vi "GetSwerveEncoders.vi"() -> (16 "Swerve 0 Velocity (ft/s)":dbl, 17 "Swerve 3 Velocity (ft/s)":dbl, 18 "Swerve 1 Velocity (ft/s)":dbl, 19 "Swerve 2 Velocity (ft/s)":dbl, 20 "Swerve 0 Azimuth Position (deg)":dbl, 21 "Swerve 0 Distance (in)":dbl, 22 "Swerve 1 Azimuth Position (deg)":dbl, 23 "Swerve 1 Distance (in)":dbl, 24 "Swerve 2 Azimuth Position (deg)":dbl, 25 "Swerve 2 Distance (in)":dbl, 26 "Swerve 3 Azimuth Position (deg)":dbl, 27 "Swerve 3 Distance (in)":dbl)   [LabVIEW 2019]
doc: "Gets the drive distance, azimuth position, and velocity encoder readings from all of the swerve modules. This VI is also useful for characterizing the drive system allowing for estimation of the robot acceleration and plotting of the module velocities. Deteremines the true shifter state based on photo-interrupter sensors on each module. Please see sensors.vi for a reading of the true robot ground speed (as this must be calculated after using the module odometry VIs)."
uses:
  9b416838-22f8-4a95-87d5-07d0cb0d5b1f.vi
  refnums.vi
  GRNF_POT.vi
  dsdata.vi
  <vilib>/Utility/xml.llb/Write to XML File(string).vi
  GRNF_CTREMotor.vi
  <vilib>/Rock Robotics/WPI/ThirdParty/Phoenix-LabVIEW/Motor Controller/Get/CTRE_Phoenix_MotorController_GetSelectedSensorData.vi
  GRNF_DI.vi
  sensors.vi
panel:
  out "Current Position (deg)":dbl
  in  "Calibrate Lamprey":T1(ring)
  out "Within Tolerance":bool
  out "Calibration Goal (deg) [0,360]":dbl format="%.2f"
  in  "Lamprey Tolerance (deg)":dbl=0.1
  in  "Calibration Step":i16
  in  "Calibration Mode":T2(ring)
  in  "Set Falcon Zero":bool
  out "Acceleration (ft/s^2)":dbl format="%.1f"
  in  "Reset Acceleration Test":bool
  in  "Plot and Measure":bool
  out "Drive Encoder Velocities (ft/s)":cluster{dbl, dbl, dbl, dbl}(graph)
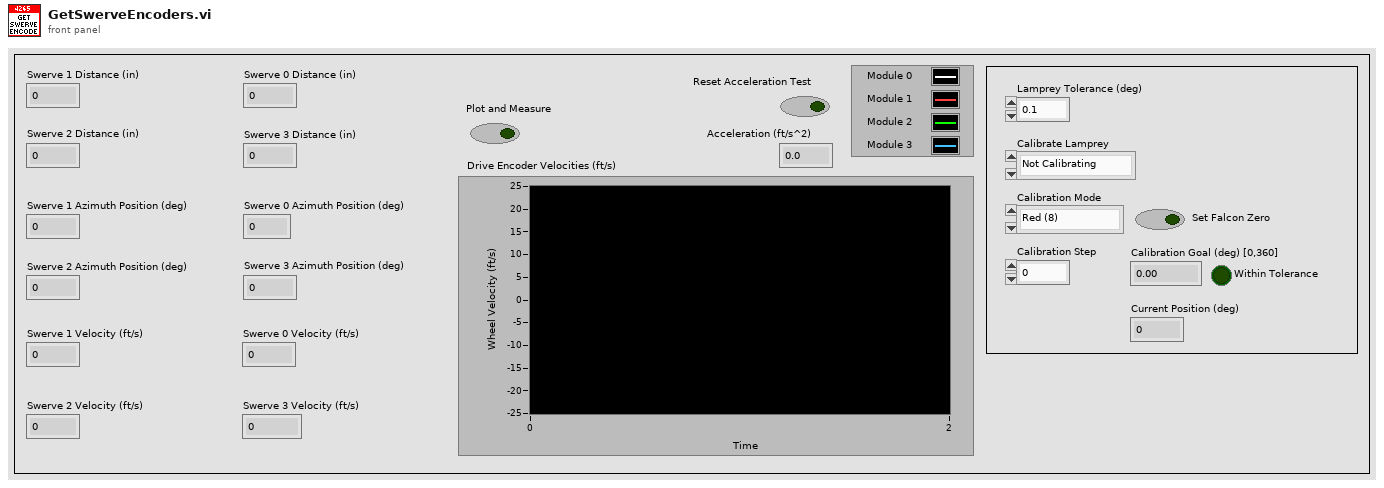
[diagram p1: front panel]
types:
  T1 = enum16{"Not Calibrating", "Module 0", "Module 1", "Module 2", "Module 3"}
  T2 = enum16{"Red (8)", "Red+Green (12)", "Red+Green+Blue (24)", "Blue (36)"}
  T3 = typedef "WPI_SwitchDevRef.ctl" = cluster{"DevStatus":errorcluster, "DIO Channel":T4, "CntIndex":T5, "Normally Closed":bool}
  T4 = typedef "FPGA_DIOChannel.ctl" = enum8{"DIO 0", "DIO 1", "DIO 2", "DIO 3", "DIO 4", "DIO 5", "DIO 6", "DIO 7", "DIO 8", "DIO 9", "DIO MXP 0", "DIO MXP 1", "DIO MXP 2", "DIO MXP 3", "DIO MXP 4", "DIO MXP 5", "DIO MXP 6", "DIO MXP 7", "DIO MXP 8", "DIO MXP 9", "DIO MXP 10", "DIO MXP 11", "DIO MXP 12", "DIO MXP 13", "DIO MXP 14", "DIO MXP 15", "SPI Port CS1", "SPI Port CS2", "SPI Port CS3", "SPI Port MISO", "SPI Port MOSI", "Invalid"}
  T5 = typedef "FPGA_CounterCtrSystemIndex.ctl" = enum8{"Ctr 0", "Ctr 1", "Ctr 2", "Ctr 3", "Ctr 4", "Ctr 5", "Ctr 6", "Ctr 7", "Invalid"}
  T6 = enum16{"Low Gear", "High Gear", "Transiting", "Unknown", "Force Low Gear"}
  T7 = typedef "WPI_MotorControlDeviceRef.ctl" = cluster{"DeviceStatus":errorcluster, "Type":T8, "PWM":cluster{"PWM Channel":T9, "DeadBand":T10}, "CAN":cluster{"Device Number":u8, "SetOutput VI Ref":variant, "GetOutput VI Ref":variant, "Enable VI Ref":variant, "Disable VI Ref":variant, "Data":variant}, "Invert":bool, "DIO PWM":cluster{"PWM \"Enable\" Channel":T9, "DIOChannel":T4, "PWM Rate":dbl}}
  T8 = typedef "WPI_MotorControlType.ctl" = enum16{"PWM", "CAN", "DIO PWM"}
  T9 = typedef "FPGA_DIOPWMChannel.ctl" = enum8{"PWM 0", "PWM 1", "PWM 2", "PWM 3", "PWM 4", "PWM 5", "PWM 6", "PWM 7", "PWM 8", "PWM 9", "PWM MXP 0", "PWM MXP 1", "PWM MXP 2", "PWM MXP 3", "PWM MXP 4", "PWM MXP 5", "PWM MXP 6", "PWM MXP 7", "PWM MXP 8", "PWM MXP 9", "Invalid"}
  T10 = typedef "WPI_PWMDeadband.ctl" = cluster{"Name":string, "maxPositivePwm":i32, "minPositivePwm":i32, "centerPwm":i32, "maxNegativePwm":i32, "minNegativePwm":i32, "angularRange":u16}
  T11 = typedef "WPI_PotentiometerDevRef.ctl" = cluster{"DevStatus":errorcluster, "Analog Channel":T12, "Invert Output":bool}
  T12 = typedef "FPGA_AIChannel.ctl" = enum8{"AI 0", "AI 1", "AI 2", "AI 3", "AI MXP 0", "AI MXP 1", "AI MXP 2", "AI MXP 3", "Invalid"}
  T13 = cluster{"Velocity (ft/s)":dbl, "Velocity (ft/s)":dbl, "Velocity (ft/s)":dbl, "Velocity (ft/s)":dbl}
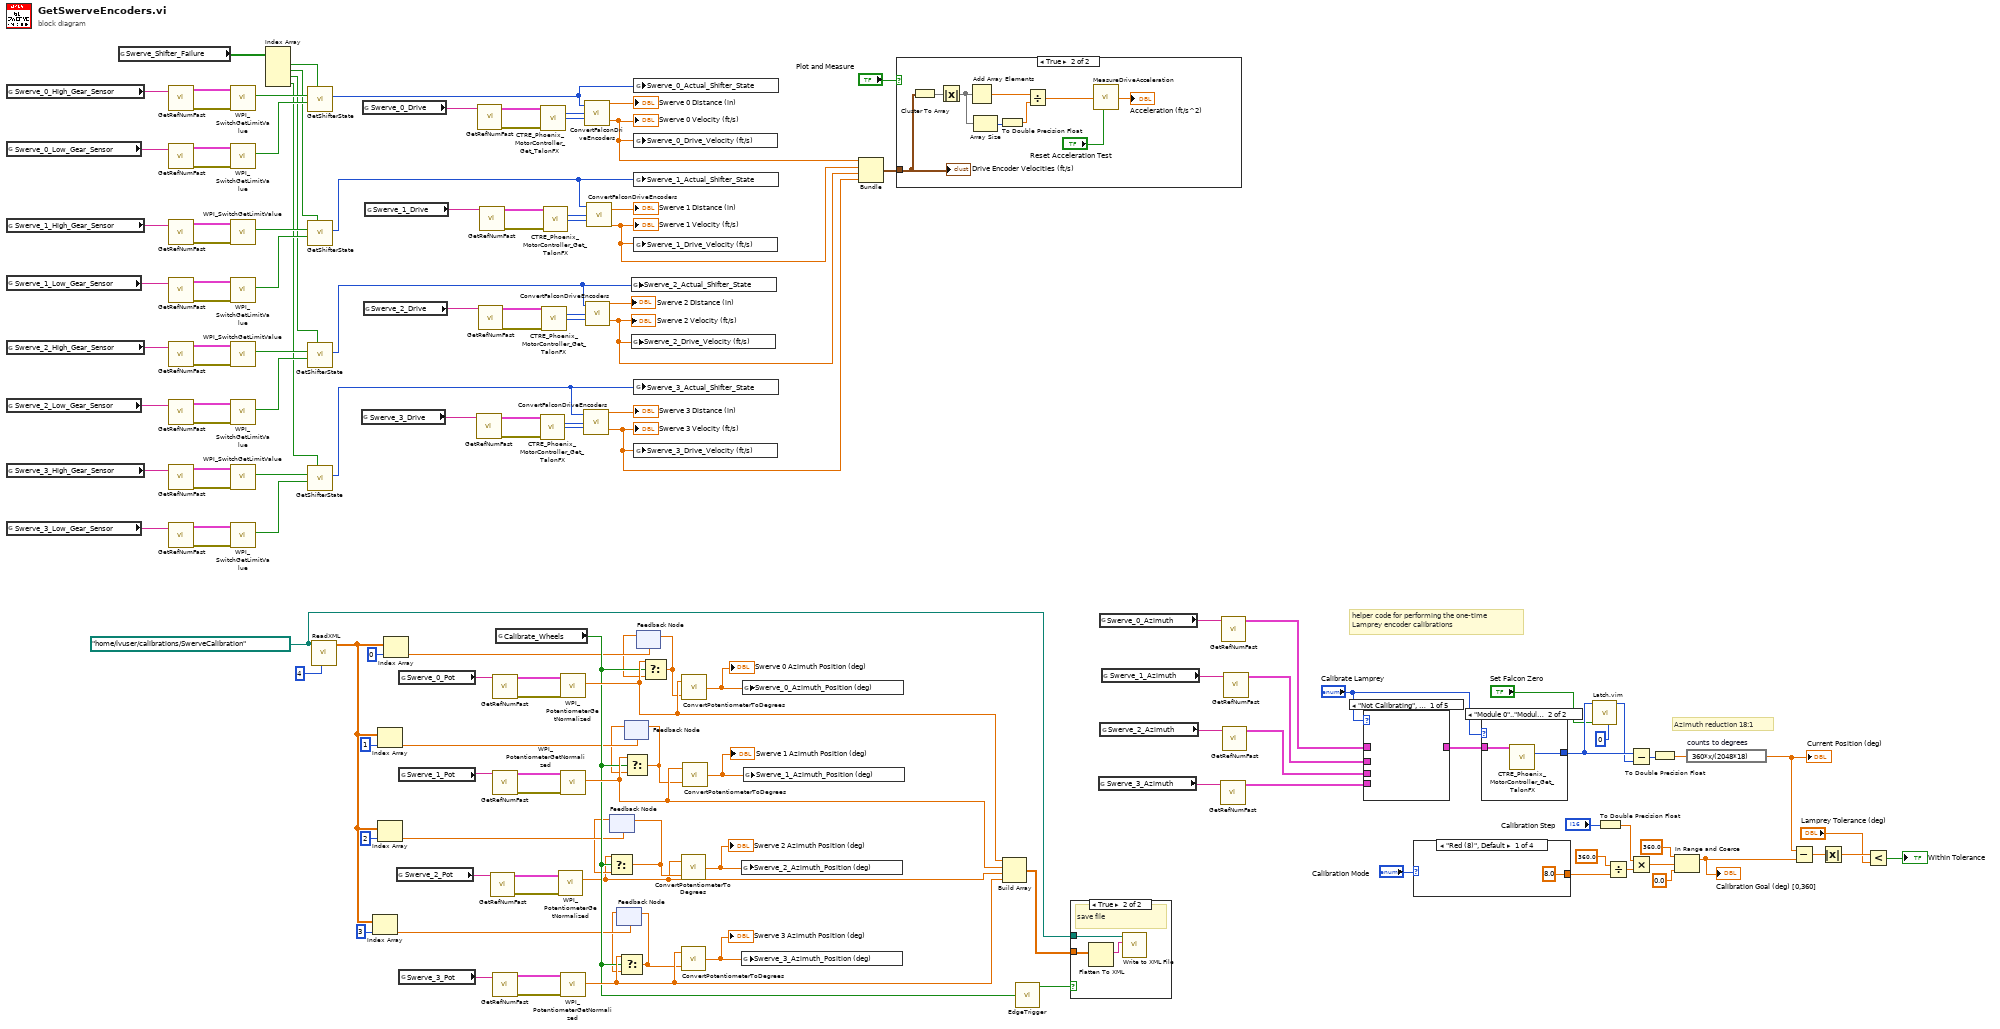
[diagram p0: block diagram]
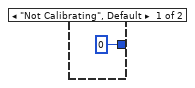
[diagram p6: hidden frame]
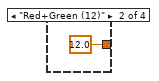
[diagram p7: hidden frame]
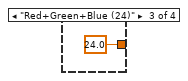
[diagram p8: hidden frame]
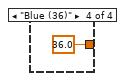
[diagram p9: hidden frame]
diagram:
  w140 = path "/home/lvuser/calibrations/SwerveCalibration" ("path")
  # "Azimuth reduction 18:1"
  # "helper code for performing the one-time\nLamprey encoder calibrations"
  n1 = global read "refnums.vi" "Swerve_0_High_Gear_Sensor"() -> (w44:string)
  n2 = global read "refnums.vi" "Swerve_0_Low_Gear_Sensor"() -> (w40:string)
  n3 = global read "refnums.vi" "Swerve_1_High_Gear_Sensor"() -> (w36:string)
  n4 = global read "refnums.vi" "Swerve_1_Low_Gear_Sensor"() -> (w32:string)
  n5 = global read "refnums.vi" "Swerve_2_High_Gear_Sensor"() -> (w27:string)
  n6 = global read "refnums.vi" "Swerve_2_Low_Gear_Sensor"() -> (w23:string)
  n7 = global read "refnums.vi" "Swerve_3_High_Gear_Sensor"() -> (w18:string)
  n8 = global read "refnums.vi" "Swerve_3_Low_Gear_Sensor"() -> (w14:string)
  n9 = global read "sensors.vi" "Swerve_Shifter_Failure"() -> (w9:bool[])
  n10 = call-poly "GetRefNumFast.vi"("RefNum Name"=w44) -> ("Error"=w42:errorcluster, "Device Reference"=w43:T3)  [unwired: 5 in]
  n11 = call-poly "GetRefNumFast.vi"("RefNum Name"=w40) -> ("Error"=w38:errorcluster, "Device Reference"=w39:T3)  [unwired: 5 in]
  n12 = call-poly "GetRefNumFast.vi"("RefNum Name"=w36) -> ("Error"=w34:errorcluster, "Device Reference"=w35:T3)  [unwired: 5 in]
  n13 = call-poly "GetRefNumFast.vi"("RefNum Name"=w32) -> ("Error"=w30:errorcluster, "Device Reference"=w31:T3)  [unwired: 5 in]
  n14 = call-poly "GetRefNumFast.vi"("RefNum Name"=w27) -> ("Error"=w25:errorcluster, "Device Reference"=w26:T3)  [unwired: 5 in]
  n15 = call-poly "GetRefNumFast.vi"("RefNum Name"=w23) -> ("Error"=w21:errorcluster, "Device Reference"=w22:T3)  [unwired: 5 in]
  n16 = call-poly "GetRefNumFast.vi"("RefNum Name"=w18) -> ("Error"=w16:errorcluster, "Device Reference"=w17:T3)  [unwired: 5 in]
  n17 = call-poly "GetRefNumFast.vi"("RefNum Name"=w14) -> ("Error"=w12:errorcluster, "Device Reference"=w13:T3)  [unwired: 5 in]
  n18 = call <vilib>:"WPI_SwitchGetLimitValue.vi"("error in (no error)"=w42, "SwitchDevRef"=w43) -> ("Switch Pressed"=w41:bool)  [unwired: 7 in, 2 out]
  n19 = call <vilib>:"WPI_SwitchGetLimitValue.vi"("error in (no error)"=w38, "SwitchDevRef"=w39) -> ("Switch Pressed"=w37:bool)  [unwired: 7 in, 2 out]
  n20 = call <vilib>:"WPI_SwitchGetLimitValue.vi"("error in (no error)"=w34, "SwitchDevRef"=w35) -> ("Switch Pressed"=w33:bool)  [unwired: 7 in, 2 out]
  n21 = call <vilib>:"WPI_SwitchGetLimitValue.vi"("error in (no error)"=w30, "SwitchDevRef"=w31) -> ("Switch Pressed"=w29:bool)  [unwired: 7 in, 2 out]
  n22 = call <vilib>:"WPI_SwitchGetLimitValue.vi"("error in (no error)"=w25, "SwitchDevRef"=w26) -> ("Switch Pressed"=w24:bool)  [unwired: 7 in, 2 out]
  n23 = call <vilib>:"WPI_SwitchGetLimitValue.vi"("error in (no error)"=w21, "SwitchDevRef"=w22) -> ("Switch Pressed"=w20:bool)  [unwired: 7 in, 2 out]
  n24 = call <vilib>:"WPI_SwitchGetLimitValue.vi"("error in (no error)"=w16, "SwitchDevRef"=w17) -> ("Switch Pressed"=w15:bool)  [unwired: 7 in, 2 out]
  n25 = call <vilib>:"WPI_SwitchGetLimitValue.vi"("error in (no error)"=w12, "SwitchDevRef"=w13) -> ("Switch Pressed"=w11:bool)  [unwired: 7 in, 2 out]
  n26 = Index Array(array=w9) -> (element #1=w8:bool, element #2=w7:bool, element #3=w6:bool, element #4=w5:bool)  [unwired: 4 in]
  n27 = call "GetShifterState.vi"("Sensor Failure"=w8, "Low Gear Sensor"=w37, "High Gear Sensor"=w41) -> ("Actual Shifter State"=w45:T6)  [unwired: 8 in]
  n28 = call "GetShifterState.vi"("Sensor Failure"=w7, "Low Gear Sensor"=w29, "High Gear Sensor"=w33) -> ("Actual Shifter State"=w28:T6)  [unwired: 8 in]
  n29 = call "GetShifterState.vi"("Sensor Failure"=w6, "Low Gear Sensor"=w20, "High Gear Sensor"=w24) -> ("Actual Shifter State"=w19:T6)  [unwired: 8 in]
  n30 = call "GetShifterState.vi"("Sensor Failure"=w5, "Low Gear Sensor"=w11, "High Gear Sensor"=w15) -> ("Actual Shifter State"=w10:T6)  [unwired: 8 in]
  n31 = call "ReadXML.vi"("Default Number of Elements"=4 ("Number of Elements"), "File Path (.xml)"=w140) -> ("Data"=w106:dbl[])  [unwired: 8 in, 1 out]
  n32 = global read "refnums.vi" "Swerve_3_Drive"() -> (w81:string)
  n33 = global read "refnums.vi" "Swerve_0_Drive"() -> (w101:string)
  n34 = global read "refnums.vi" "Swerve_2_Drive"() -> (w88:string)
  n35 = global read "refnums.vi" "Swerve_1_Drive"() -> (w93:string)
  n36 = Index Array(array=w106, index=3) -> (element=w124:dbl)
  n37 = Index Array(array=w106, index=1) -> (element=w129:dbl)
  n38 = Index Array(array=w106, index=2) -> (element=w126:dbl)
  n39 = Index Array(array=w106, index=0) -> (element=w132:dbl)
  n40 = global read "refnums.vi" "Swerve_2_Pot"() -> (w110:string)
  n41 = global read "refnums.vi" "Swerve_0_Pot"() -> (w118:string)
  n42 = global read "refnums.vi" "Swerve_1_Pot"() -> (w113:string)
  n43 = global read "refnums.vi" "Swerve_3_Pot"() -> (w109:string)
  n44 = call-poly "GetRefNumFast.vi"("RefNum Name"=w81) -> ("Error"=w83:errorcluster, "Device Reference"=w82:T7)  [unwired: 5 in]
  n45 = call-poly "GetRefNumFast.vi"("RefNum Name"=w101) -> ("Error"=w103:errorcluster, "Device Reference"=w102:T7)  [unwired: 5 in]
  n46 = call-poly "GetRefNumFast.vi"("RefNum Name"=w88) -> ("Error"=w2:errorcluster, "Device Reference"=w1:T7)  [unwired: 5 in]
  n47 = call-poly "GetRefNumFast.vi"("RefNum Name"=w93) -> ("Error"=w95:errorcluster, "Device Reference"=w94:T7)  [unwired: 5 in]
  n48 = call-poly "GetRefNumFast.vi"("RefNum Name"=w110) -> ("Error"=w111:errorcluster, "Device Reference"=w112:T11)  [unwired: 5 in]
  n49 = call-poly "GetRefNumFast.vi"("RefNum Name"=w118) -> ("Error"=w116:errorcluster, "Device Reference"=w117:T11)  [unwired: 5 in]
  n50 = call-poly "GetRefNumFast.vi"("RefNum Name"=w113) -> ("Error"=w114:errorcluster, "Device Reference"=w115:T11)  [unwired: 5 in]
  n51 = call-poly "GetRefNumFast.vi"("RefNum Name"=w109) -> ("Error"=w107:errorcluster, "Device Reference"=w108:T11)  [unwired: 5 in]
  n52 = global read "dsdata.vi" "Calibrate_Wheels"() -> (w139:bool)
  n53 = call-poly <vilib>:"CTRE_Phoenix_MotorController_Get_TalonFX.vi"("PhoenixMotorControlDevRef"=w82, "error in"=w83) -> ("Position (Raw Sensor Units)"=w79:i32, "Velocity (Raw Sensor Units per 100 ms)"=w80:i32)  [unwired: 10 in, 2 out]
  n54 = call-poly <vilib>:"CTRE_Phoenix_MotorController_Get_TalonFX.vi"("PhoenixMotorControlDevRef"=w102, "error in"=w103) -> ("Position (Raw Sensor Units)"=w96:i32, "Velocity (Raw Sensor Units per 100 ms)"=w97:i32)  [unwired: 10 in, 2 out]
  n55 = call-poly <vilib>:"CTRE_Phoenix_MotorController_Get_TalonFX.vi"("PhoenixMotorControlDevRef"=w1, "error in"=w2) -> ("Position (Raw Sensor Units)"=w86:i32, "Velocity (Raw Sensor Units per 100 ms)"=w87:i32)  [unwired: 10 in, 2 out]
  n56 = call-poly <vilib>:"CTRE_Phoenix_MotorController_Get_TalonFX.vi"("PhoenixMotorControlDevRef"=w94, "error in"=w95) -> ("Position (Raw Sensor Units)"=w91:i32, "Velocity (Raw Sensor Units per 100 ms)"=w92:i32)  [unwired: 10 in, 2 out]
  n57 = call <vilib>:"WPI_PotentiometerGetNormalized.vi"("error in"=w111, "PotDevRef"=w112) -> ("Normalized Value"=w3:dbl)  [unwired: 7 in, 2 out]
  n58 = call <vilib>:"WPI_PotentiometerGetNormalized.vi"("error in"=w116, "PotDevRef"=w117) -> ("Normalized Value"=w141:dbl)  [unwired: 7 in, 2 out]
  n59 = call <vilib>:"WPI_PotentiometerGetNormalized.vi"("error in"=w114, "PotDevRef"=w115) -> ("Normalized Value"=w143:dbl)  [unwired: 7 in, 2 out]
  n60 = call <vilib>:"WPI_PotentiometerGetNormalized.vi"("error in"=w107, "PotDevRef"=w108) -> ("Normalized Value"=w142:dbl)  [unwired: 7 in, 2 out]
  n61 = call "ConvertFalconDriveEncoders.vi"("Velocity (Raw Sensor Units per 100 ms)"=w80, "Distance (Raw Sensor Units)"=w79, "Shifter State"=w10) -> ("Velocity (ft/s)"=w77:dbl, "Distance (in)"=→"Swerve 3 Distance (in)":dbl)
  "Swerve 3 Velocity (ft/s)" <- w77
  n62 = call "ConvertFalconDriveEncoders.vi"("Velocity (Raw Sensor Units per 100 ms)"=w97, "Distance (Raw Sensor Units)"=w96, "Shifter State"=w45) -> ("Velocity (ft/s)"=w99:dbl, "Distance (in)"=→"Swerve 0 Distance (in)":dbl)
  "Swerve 0 Velocity (ft/s)" <- w99
  n63 = call "ConvertFalconDriveEncoders.vi"("Velocity (Raw Sensor Units per 100 ms)"=w87, "Distance (Raw Sensor Units)"=w86, "Shifter State"=w19) -> ("Velocity (ft/s)"=w84:dbl, "Distance (in)"=→"Swerve 2 Distance (in)":dbl)
  "Swerve 2 Velocity (ft/s)" <- w84
  n64 = call "ConvertFalconDriveEncoders.vi"("Velocity (Raw Sensor Units per 100 ms)"=w92, "Distance (Raw Sensor Units)"=w91, "Shifter State"=w28) -> ("Velocity (ft/s)"=w89:dbl, "Distance (in)"=→"Swerve 1 Distance (in)":dbl)
  "Swerve 1 Velocity (ft/s)" <- w89
  n65 = feedback #1(w126) -> (w125:dbl)
  n66 = Select(t=w3, s=w139, f=w125) -> (s? t:f=w4:dbl)
  n67 = feedback-in #1(w4) -> ()
  n68 = feedback #2(w124) -> (w123:dbl)
  n69 = Select(t=w142, s=w139, f=w123) -> (s? t:f=w119:dbl)
  n70 = feedback-in #2(w119) -> ()
  n71 = feedback #3(w129) -> (w128:dbl)
  n72 = Select(t=w143, s=w139, f=w128) -> (s? t:f=w120:dbl)
  n73 = feedback-in #3(w120) -> ()
  n74 = global write "sensors.vi" "Swerve_2_Actual_Shifter_State"(w19) -> ()
  n75 = global write "sensors.vi" "Swerve_2_Drive_Velocity (ft/s)"(w84) -> ()
  n76 = global write "sensors.vi" "Swerve_0_Actual_Shifter_State"(w45) -> ()
  n77 = global write "sensors.vi" "Swerve_0_Drive_Velocity (ft/s)"(w99) -> ()
  n78 = global write "sensors.vi" "Swerve_1_Actual_Shifter_State"(w28) -> ()
  n79 = global write "sensors.vi" "Swerve_1_Drive_Velocity (ft/s)"(w89) -> ()
  n80 = global write "sensors.vi" "Swerve_3_Actual_Shifter_State"(w10) -> ()
  n81 = global write "sensors.vi" "Swerve_3_Drive_Velocity (ft/s)"(w77) -> ()
  n82 = feedback #4(w132) -> (w131:dbl)
  n83 = Select(t=w141, s=w139, f=w131) -> (s? t:f=w121:dbl)
  n84 = feedback-in #4(w121) -> ()
  n85 = call "ConvertPotentiometerToDegrees.vi"("Zero Position [0-1]"=w4, "Raw Potentiometer Value [0,1]"=w3) -> ("Orientation (deg) [-180,+180]"=w135:dbl)
  "Swerve 2 Azimuth Position (deg)" <- w135
  n86 = call "ConvertPotentiometerToDegrees.vi"("Zero Position [0-1]"=w119, "Raw Potentiometer Value [0,1]"=w142) -> ("Orientation (deg) [-180,+180]"=w134:dbl)
  "Swerve 3 Azimuth Position (deg)" <- w134
  n87 = call "ConvertPotentiometerToDegrees.vi"("Zero Position [0-1]"=w121, "Raw Potentiometer Value [0,1]"=w141) -> ("Orientation (deg) [-180,+180]"=w137:dbl)
  "Swerve 0 Azimuth Position (deg)" <- w137
  n88 = call "ConvertPotentiometerToDegrees.vi"("Zero Position [0-1]"=w120, "Raw Potentiometer Value [0,1]"=w143) -> ("Orientation (deg) [-180,+180]"=w136:dbl)
  "Swerve 1 Azimuth Position (deg)" <- w136
  n89 = global write "sensors.vi" "Swerve_2_Azimuth_Position (deg)"(w135) -> ()
  n90 = global write "sensors.vi" "Swerve_3_Azimuth_Position (deg)"(w134) -> ()
  n91 = global write "sensors.vi" "Swerve_0_Azimuth_Position (deg)"(w137) -> ()
  n92 = global write "sensors.vi" "Swerve_1_Azimuth_Position (deg)"(w136) -> ()
  n93 = Bundle("Velocity (ft/s)"=w99, "Velocity (ft/s)"=w89, "Velocity (ft/s)"=w84, "Velocity (ft/s)"=w77) -> (w98:T13)  [unwired: 1 in]
  n94 = case shown="True" "Plot and Measure" {
    tunnel: w98 -> [_ w148]
    frame False {
    }
    frame True {
      n95 = Cluster To Array(cluster=w148) -> (array=w150:dbl[])
      n96 = Absolute Value(x=w150) -> (abs(x)=w153:dbl[])
      n97 = Add Array Elements(numeric array=w153) -> (sum=w149:dbl)
      n98 = Array Size(array=w153) -> (size(s)=w151:i32)
      n99 = To Double Precision Float(number=w151) -> (double precision float=w152:dbl)
      n100 = Divide(x=w149, y=w152) -> (x/y=w147:dbl)
      n101 = call "MeasureDriveAcceleration.vi"("Average Drive Velocity (ft/s)"=w147, "Reset"="Reset Acceleration Test") -> ("Acceleration (ft/s^2)"=→"Acceleration (ft/s^2)":dbl)  [unwired: 3 in]
      "Drive Encoder Velocities (ft/s)" <- w148
    }
  }
  n102 = Build Array(w141, w143, w3, w142) -> (w144:dbl[])
  n103 = call "EdgeTrigger.vi"("Input Signal"=w139) -> ("Rising Edge Trigger"=w138:bool)  [unwired: 2 out]
  n104 = case shown="True" w138 {
    tunnel: w140 -> [_ w156]
    tunnel: w144 -> [_ w155]
    frame False {
    }
    frame True {
      # "save file"
      n105 = Flatten To XML(anything=w155) -> (xml string=w154:string)
      n106 = call-poly <vilib>:"Write to XML File.vi"("XML Input"=w154, "XML File Path"=w156) -> ()  [unwired: 7 in, 3 out]
    }
  }
  n107 = global read "refnums.vi" "Swerve_3_Azimuth"() -> (w50:string)
  n108 = global read "refnums.vi" "Swerve_0_Azimuth"() -> (w53:string)
  n109 = global read "refnums.vi" "Swerve_2_Azimuth"() -> (w51:string)
  n110 = global read "refnums.vi" "Swerve_1_Azimuth"() -> (w52:string)
  n111 = call-poly "GetRefNumFast.vi"("RefNum Name"=w50) -> ("Device Reference"=w46:T7)  [unwired: 5 in, 1 out]
  n112 = call-poly "GetRefNumFast.vi"("RefNum Name"=w53) -> ("Device Reference"=w49:T7)  [unwired: 5 in, 1 out]
  n113 = call-poly "GetRefNumFast.vi"("RefNum Name"=w51) -> ("Device Reference"=w47:T7)  [unwired: 5 in, 1 out]
  n114 = call-poly "GetRefNumFast.vi"("RefNum Name"=w52) -> ("Device Reference"=w48:T7)  [unwired: 5 in, 1 out]
  n115 = case shown="\"Not Calibrating\", Default" "Calibrate Lamprey" {
    tunnel: [_ w157 w158 w159 w160] -> w59
    tunnel: w49 -> [_ w157 _ _ _]
    tunnel: w48 -> [_ _ w158 _ _]
    tunnel: w47 -> [_ _ _ w159 _]
    tunnel: w46 -> [_ _ _ _ w160]
    frame "Not Calibrating", Default {
    }
    frame "Module 0" {
    }
    frame "Module 1" {
    }
    frame "Module 2" {
    }
    frame "Module 3" {
    }
  }
  n116 = case shown="\"Red (8)\", Default" "Calibration Mode" {
    tunnel: [8.0 12.0 24.0 36.0] -> w73
    frame "Red (8)", Default {
    }
    frame "Red+Green (12)" {
    }
    frame "Red+Green+Blue (24)" {
    }
    frame "Blue (36)" {
    }
  }
  n117 = case shown="\"Module 0\"..\"Module 3\"" "Calibrate Lamprey" {
    tunnel: [0 ("Position (Raw Sensor Units)") w167] -> w57
    tunnel: w59 -> [_ w166]
    frame "Not Calibrating", Default {
    }
    frame "Module 0".."Module 3" {
      n118 = call-poly <vilib>:"CTRE_Phoenix_MotorController_Get_TalonFX.vi"("PhoenixMotorControlDevRef"=w166) -> ("Position (Raw Sensor Units)"=w167:i32)  [unwired: 11 in, 3 out]
    }
  }
  n119 = call "Latch.vim"("Default Value"=0, "Latch Signal"="Set Falcon Zero", "Latch Value"=w57) -> ("Latched"=w56:i32)  [unwired: 8 in]
  n120 = To Double Precision Float(number="Calibration Step") -> (double precision float=w70:dbl)
  n121 = Divide(x=360.0, y=w73) -> (x/y=w71:dbl)
  n122 = Subtract(x=w57, y=w56) -> (x-y=w76:i32)
  n123 = Multiply(x=w70, y=w71) -> (x*y=w69:dbl)
  n124 = To Double Precision Float(number=w76) -> (double precision float=w75:dbl)
  n125 = In Range and Coerce(upper limit=360.0, x=w69, lower limit=0.0) -> (coerced(x)=w65:dbl)  [unwired: 1 out]
  "Calibration Goal (deg) [0,360]" <- w65
  n126 = expression code="360*x/(2048*18)" "counts to degrees"(w75) -> (w64:dbl)
  "Current Position (deg)" <- w64
  n127 = Subtract(x=w64, y=w65) -> (x-y=w63:dbl)
  n128 = Absolute Value(x=w63) -> (abs(x)=w62:dbl)
  n129 = Less?(x=w62, y="Lamprey Tolerance (deg)") -> (x < y?=→"Within Tolerance":bool)
